vi "CHK_CRC.vi"(1 "data in":string) -> (0 "Valid?!":bool, 2 "CRC-Bytes":string)   [LabVIEW 2013]
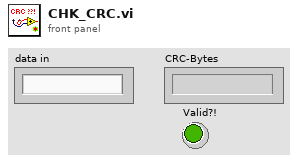
[diagram p1: front panel]
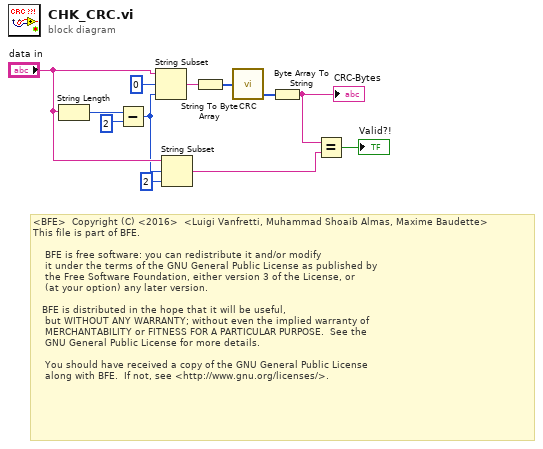
[diagram p0: block diagram]
diagram:
  # "<BFE>  Copyright (C) <2016>  <Luigi Vanfretti, Muhammad Shoaib Almas, Maxime Baudette> \nThis file is part of BFE.\n\n    BFE is free software: you can redistribute it and/or modify\n    it under the terms of the GNU General Public License as published by\n    the Free Software Foundation, either version 3 of the License, or\n    (at your option) any later version.\n\n   BFE is distributed in the hope that it will be useful,\n    but WITHOUT ANY WARRANTY; without even the implied warranty of\n    MERCHANTABILITY or FITNESS FOR A PARTICULAR PURPOSE.  See the\n    GNU General Public License for more details.\n\n    You should have received a copy of the GNU General Public License\n    along with BFE.  If not, see <http://www.gnu.org/licenses/>."
  n1 = String Length(string="data in") -> (length=w8:i32)
  n2 = Subtract(x=w8, y=2) -> (x-y=w5:i32)
  n3 = String Subset(string="data in", offset (0)=0, length (rest)=w5) -> (substring=w10:string)
  n4 = String Subset(string="data in", offset (0)=w5, length (rest)=2 ("length (rest)")) -> (substring=w2:string)
  n5 = String To Byte Array(string=w10) -> (unsigned byte array=w11:u8[])
  n6 = call "CRC.vi"("byte array"=w11) -> ("CRCbytes"=w12:u8[])  [unwired: 1 out]
  n7 = Byte Array To String(unsigned byte array=w12) -> (string=w3:string)
  "CRC-Bytes" <- w3
  n8 = Equal?(x=w3, y=w2) -> (x = y?=→"Valid?!":bool)
